vi "Configure Edge Trigger.vi"(0 "VISA resource name":refnum<visa-resource-name>, 5 "Trigger Source (1: Channel 1)":u16(ring)=1 items=["Channel 1"=1, "Channel 2"=2], 7 "Trigger Slope (0: Rising)":u16(ring) items=["Rising", "Falling"], 9 "Trigger Level (0.0 V)":dbl, 11 "error in (no error)":errorcluster) -> (4 "VISA resource name out":refnum<visa-resource-name>, 15 "error out":errorcluster)   [LabVIEW 2020, in "Template - Scope.lvlib"]
doc: "Configures edge trigger settings. An edge trigger occurs when the trigger signal passes through the voltage threshold that you specify with the <B>Trigger Level</B> control and has the slope that you specify with the <B>Trigger Slope</B> control."
uses:
  <instrlib>/_Template - Scope/Template - Scope.lvlib
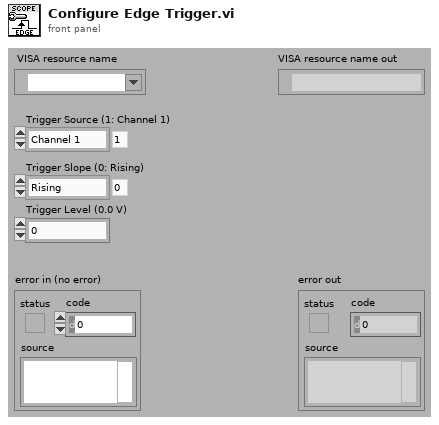
[diagram p1: front panel]
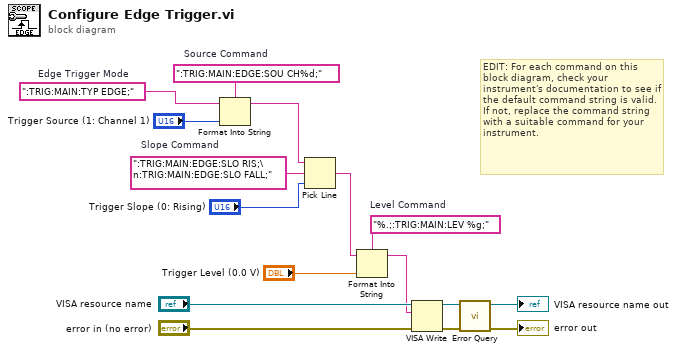
[diagram p0: block diagram]
diagram:
  w5 = ":TRIG:MAIN:EDGE:SLO RIS;\n:TRIG:MAIN:EDGE:SLO FALL;"  # Slope Command
  w7 = "%.;:TRIG:MAIN:LEV %g;"  # Level Command
  w8 = ":TRIG:MAIN:TYP EDGE;"  # Edge Trigger Mode
  w10 = ":TRIG:MAIN:EDGE:SOU CH%d;"  # Source Command
  # "EDIT: For each command on this block diagram, check your instrument's documentation to see if the default command string is valid.  If not, replace the command string with a suitable command for your instrument."
  n1 = Format Into String(format string=w10, initial string=w8, "Trigger Source (1: Channel 1)") -> (resulting string=w2:string)  [unwired: 1 in, 1 out]
  n2 = Pick Line(string ("")=w2, multi-line string=w5, line index="Trigger Slope (0: Rising)") -> (output string=w1:string)
  n3 = Format Into String(format string=w7, initial string=w1, "Trigger Level (0.0 V)") -> (resulting string=w3:string)  [unwired: 1 in, 1 out]
  n4 = VISA Write(VISA resource name="VISA resource name", write buffer=w3, error in (no error)="error in (no error)") -> (VISA resource name out=w12:refnum<visa-resource-name>, error out=w11:errorcluster)  [unwired: 1 out]
  n5 = call <instrlib>:"Error Query.vi"("error in (no error)"=w11, "VISA resource name"=w12) -> ("error out"=→"error out":errorcluster, "VISA resource name out"=→"VISA resource name out":refnum<visa-resource-name>)  [unwired: 6 in, 2 out]
